vi "CameraSerial_Demo_Legacy.vi"() -> (4 "图像时间戳":u32=16532020 format="%_32g")   [LabVIEW 2015]
uses:
  F:/labview/labview2014 NI/LabVIEW 2015/examples/Instrument IO/Serial/support/Serial - Settings.ctl
  <vilib>/Instr/_visa.llb/VISA Configure Serial Port (Instr).vi
  MVCAMSDK.dll
  <vilib>/Analysis/NI_AALBase.lvlib
panel:
  in  "停止":bool
  out "信号曲线":cluster{dbl[], dbl[]}(graph)
  in  "串口设置":T1={"波特率"=9600, "数据比特"=8, "奇偶"=enum."None", "停止位"=10, "流控制"=0} {"流控制" items=["无"=0, "XON/XOFF"=1, "RTS/CTS"=2, "DTR/DSR"=4]; "停止位" items=["1.0"=10, "1.5"=15, "2.0"=20]; "数据比特" min=5 max=8 step=1; "波特率" items=["75"=75, "110"=110, "134"=134, "150"=150, "300"=300, "600"=600, "1200"=1200, "1800"=1800, "2400"=2400, "4800"=4800, "7200"=7200, "9600"=9600, "14400"=14400, "19200"=19200, "28800"=28800, "38400"=38400, "56000"=56000, "57600"=57600, "115200"=115200, "128000"=128000, "230400"=230400]}
  in  "VISA资源名称":refnum<visa-resource-name>="COM3"
  out "variance 2":dbl caption="方差2" format="%0.3e"
  out "光强图 2":u64[](graph)
  out "variance":dbl caption="方差" format="%0.3e"
  out "相机图像":T2(plugin-control)
  out "光强图":u64[](graph)
  in  "自定义分辨率设置":bool
  in  "预设分辨率设置":bool
  out "帧速":u32
  out "帧间耗时\n单位：（0.1ms）":u32
  in  "相机枚举":T3(ring)
  in  "自动曝光模式":bool=TRUE caption="软触发"
  in  "手动曝光模式":bool caption="软触发"
  in  "硬触发模式":bool caption="软触发"
  in  "软触发模式":bool caption="软触发"
  in  "连续模式":bool caption="软触发"
  in  "软触发一帧":bool caption="软触发"
  in  "读取自定义数据":bool
  in  "写入自定义数据":bool
  in  "拍照":bool
  in  "相机参数":bool=TRUE
  in  "Stop":bool
  in  "激活预览":bool=TRUE
  out "Image":T2(plugin-control)
  # "写入自定义数据"
  # "相机原生分辨率设置"
  # "触发设置"
  # "曝光设置"
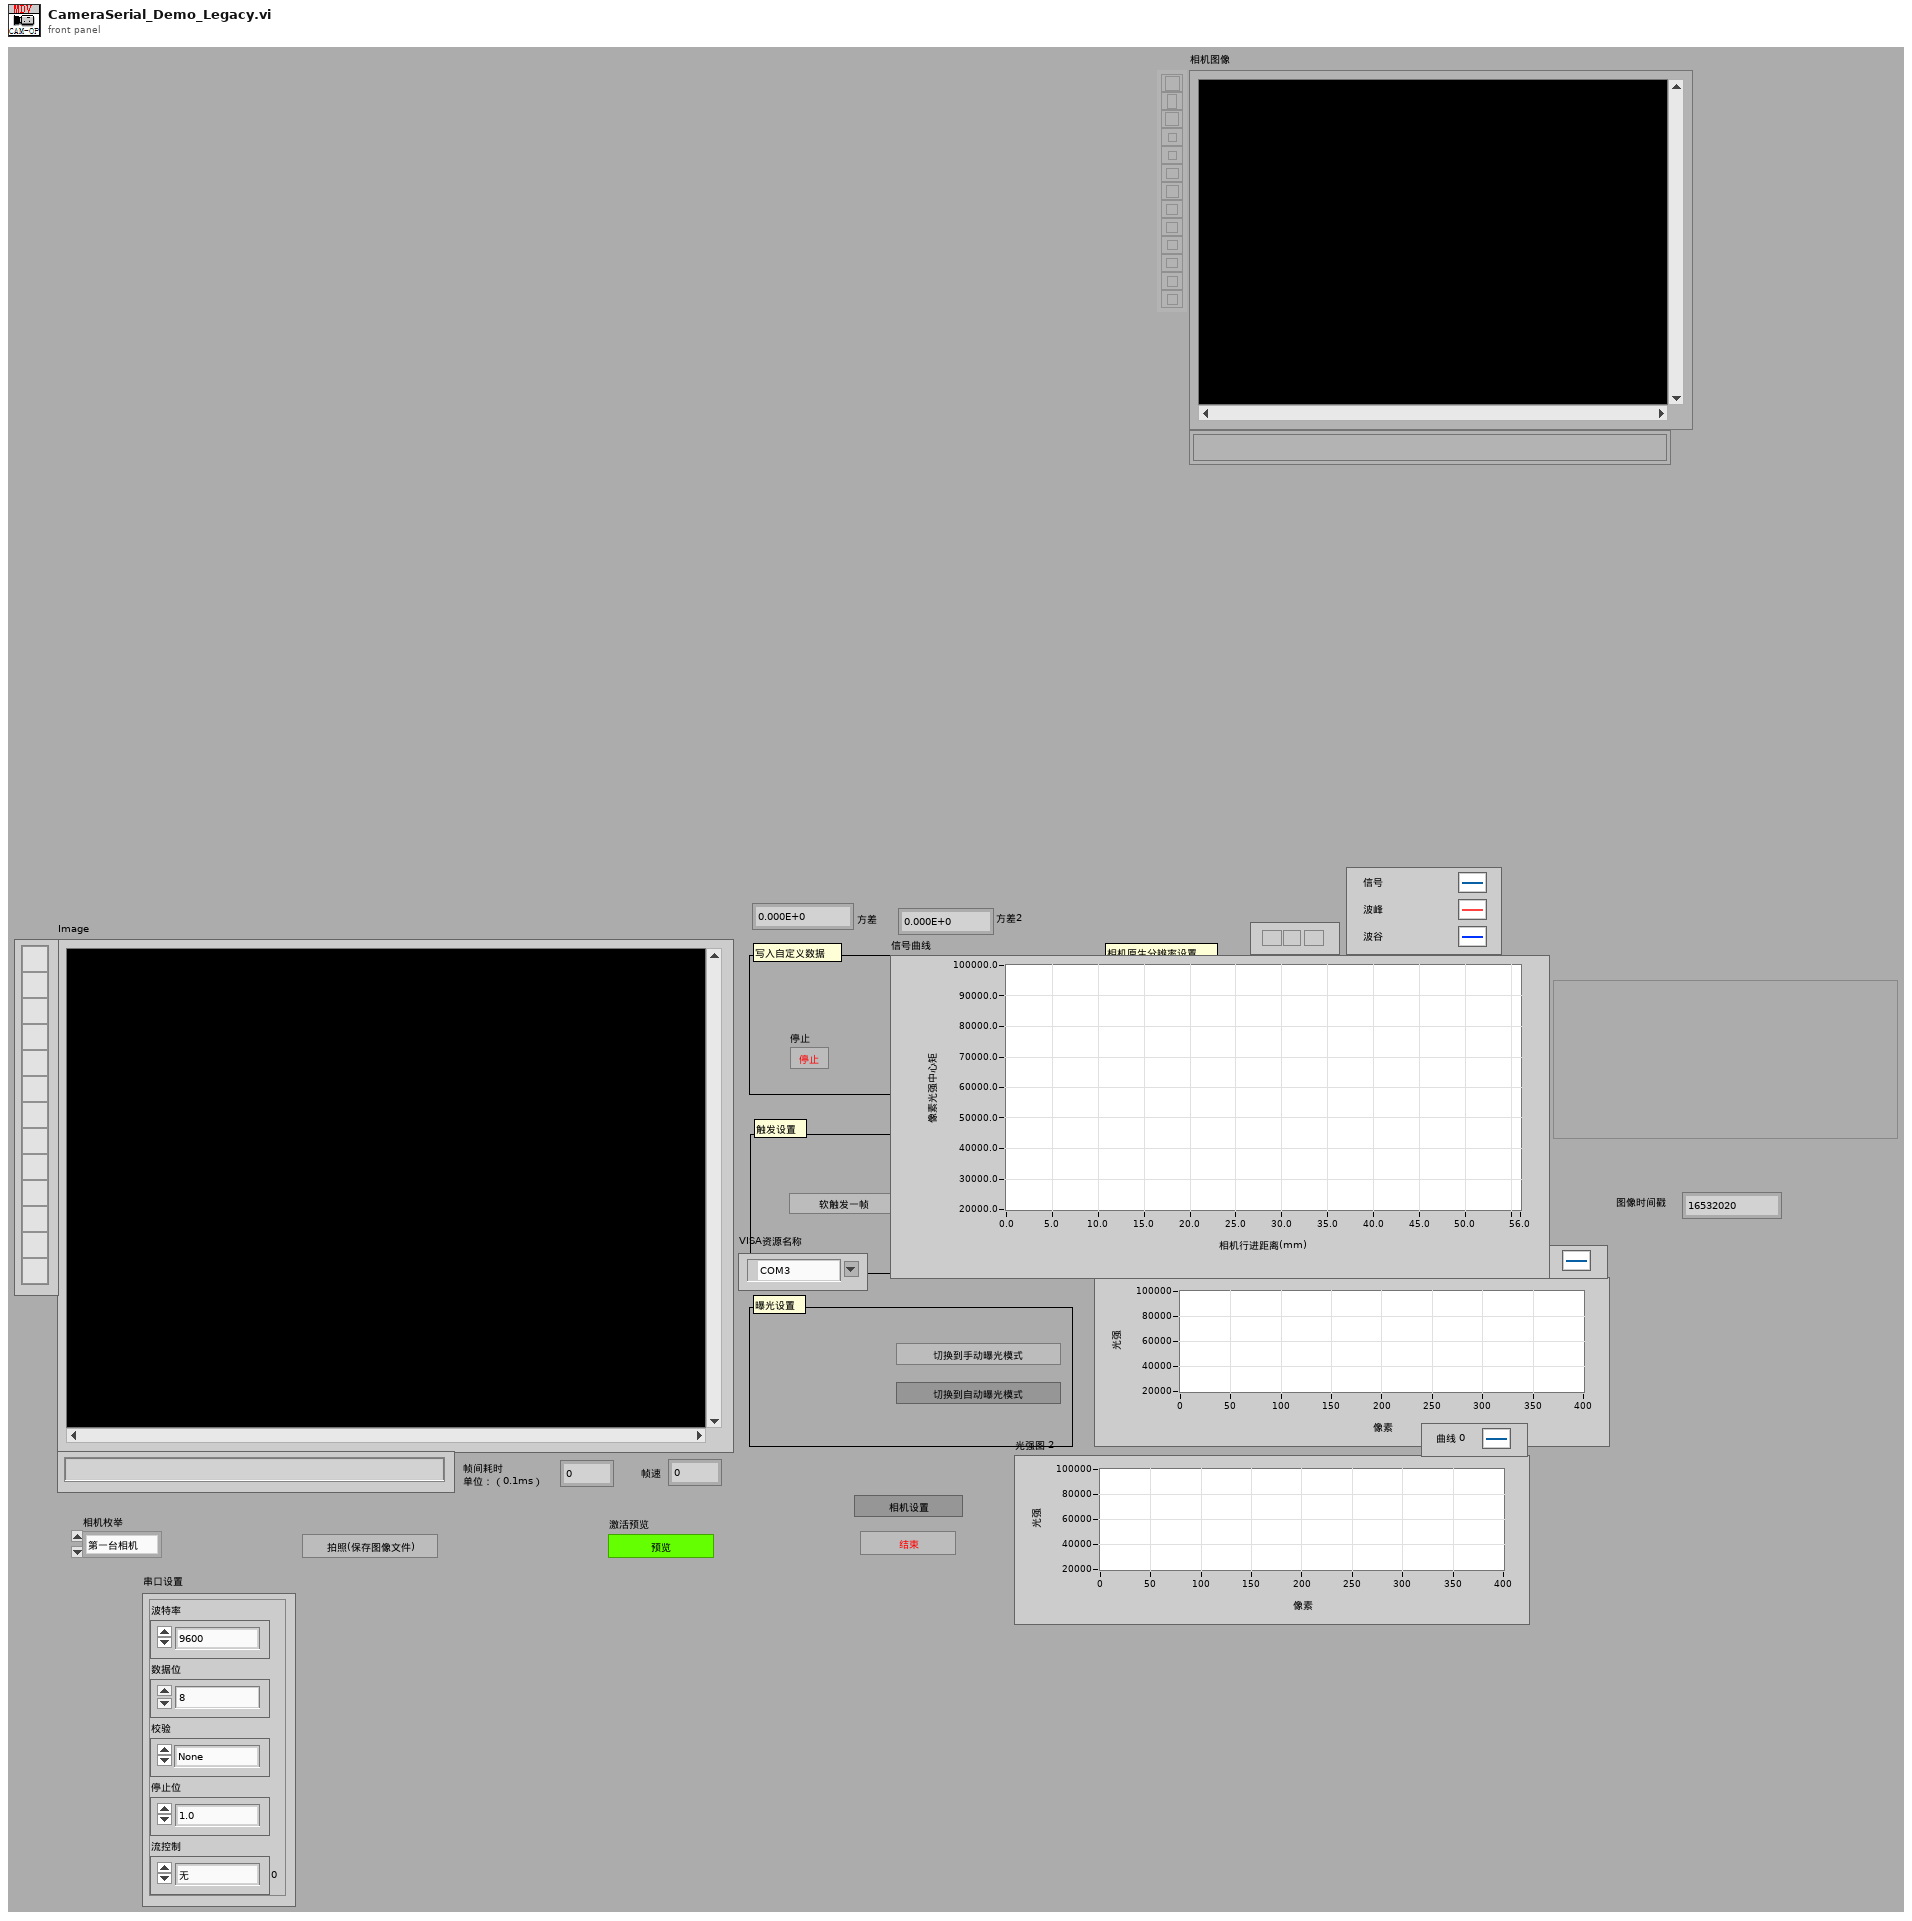
[diagram p1: front panel]
types:
  T1 = typedef "Serial - Settings.ctl" = cluster{"波特率":u32, "数据比特":u16, "奇偶":enum16{"None", "Odd", "Even", "Mark", "Space"}, "停止位":u16, "流控制":u16}
  T2 = typedef "IMAQ Image.ctl" = refnum<image>
  T3 = enum16{"第一台相机", "第二台相机", "第三台相机", "第四台相机", "第五台相机"}
  T4 = typedef "Image Type" = u32
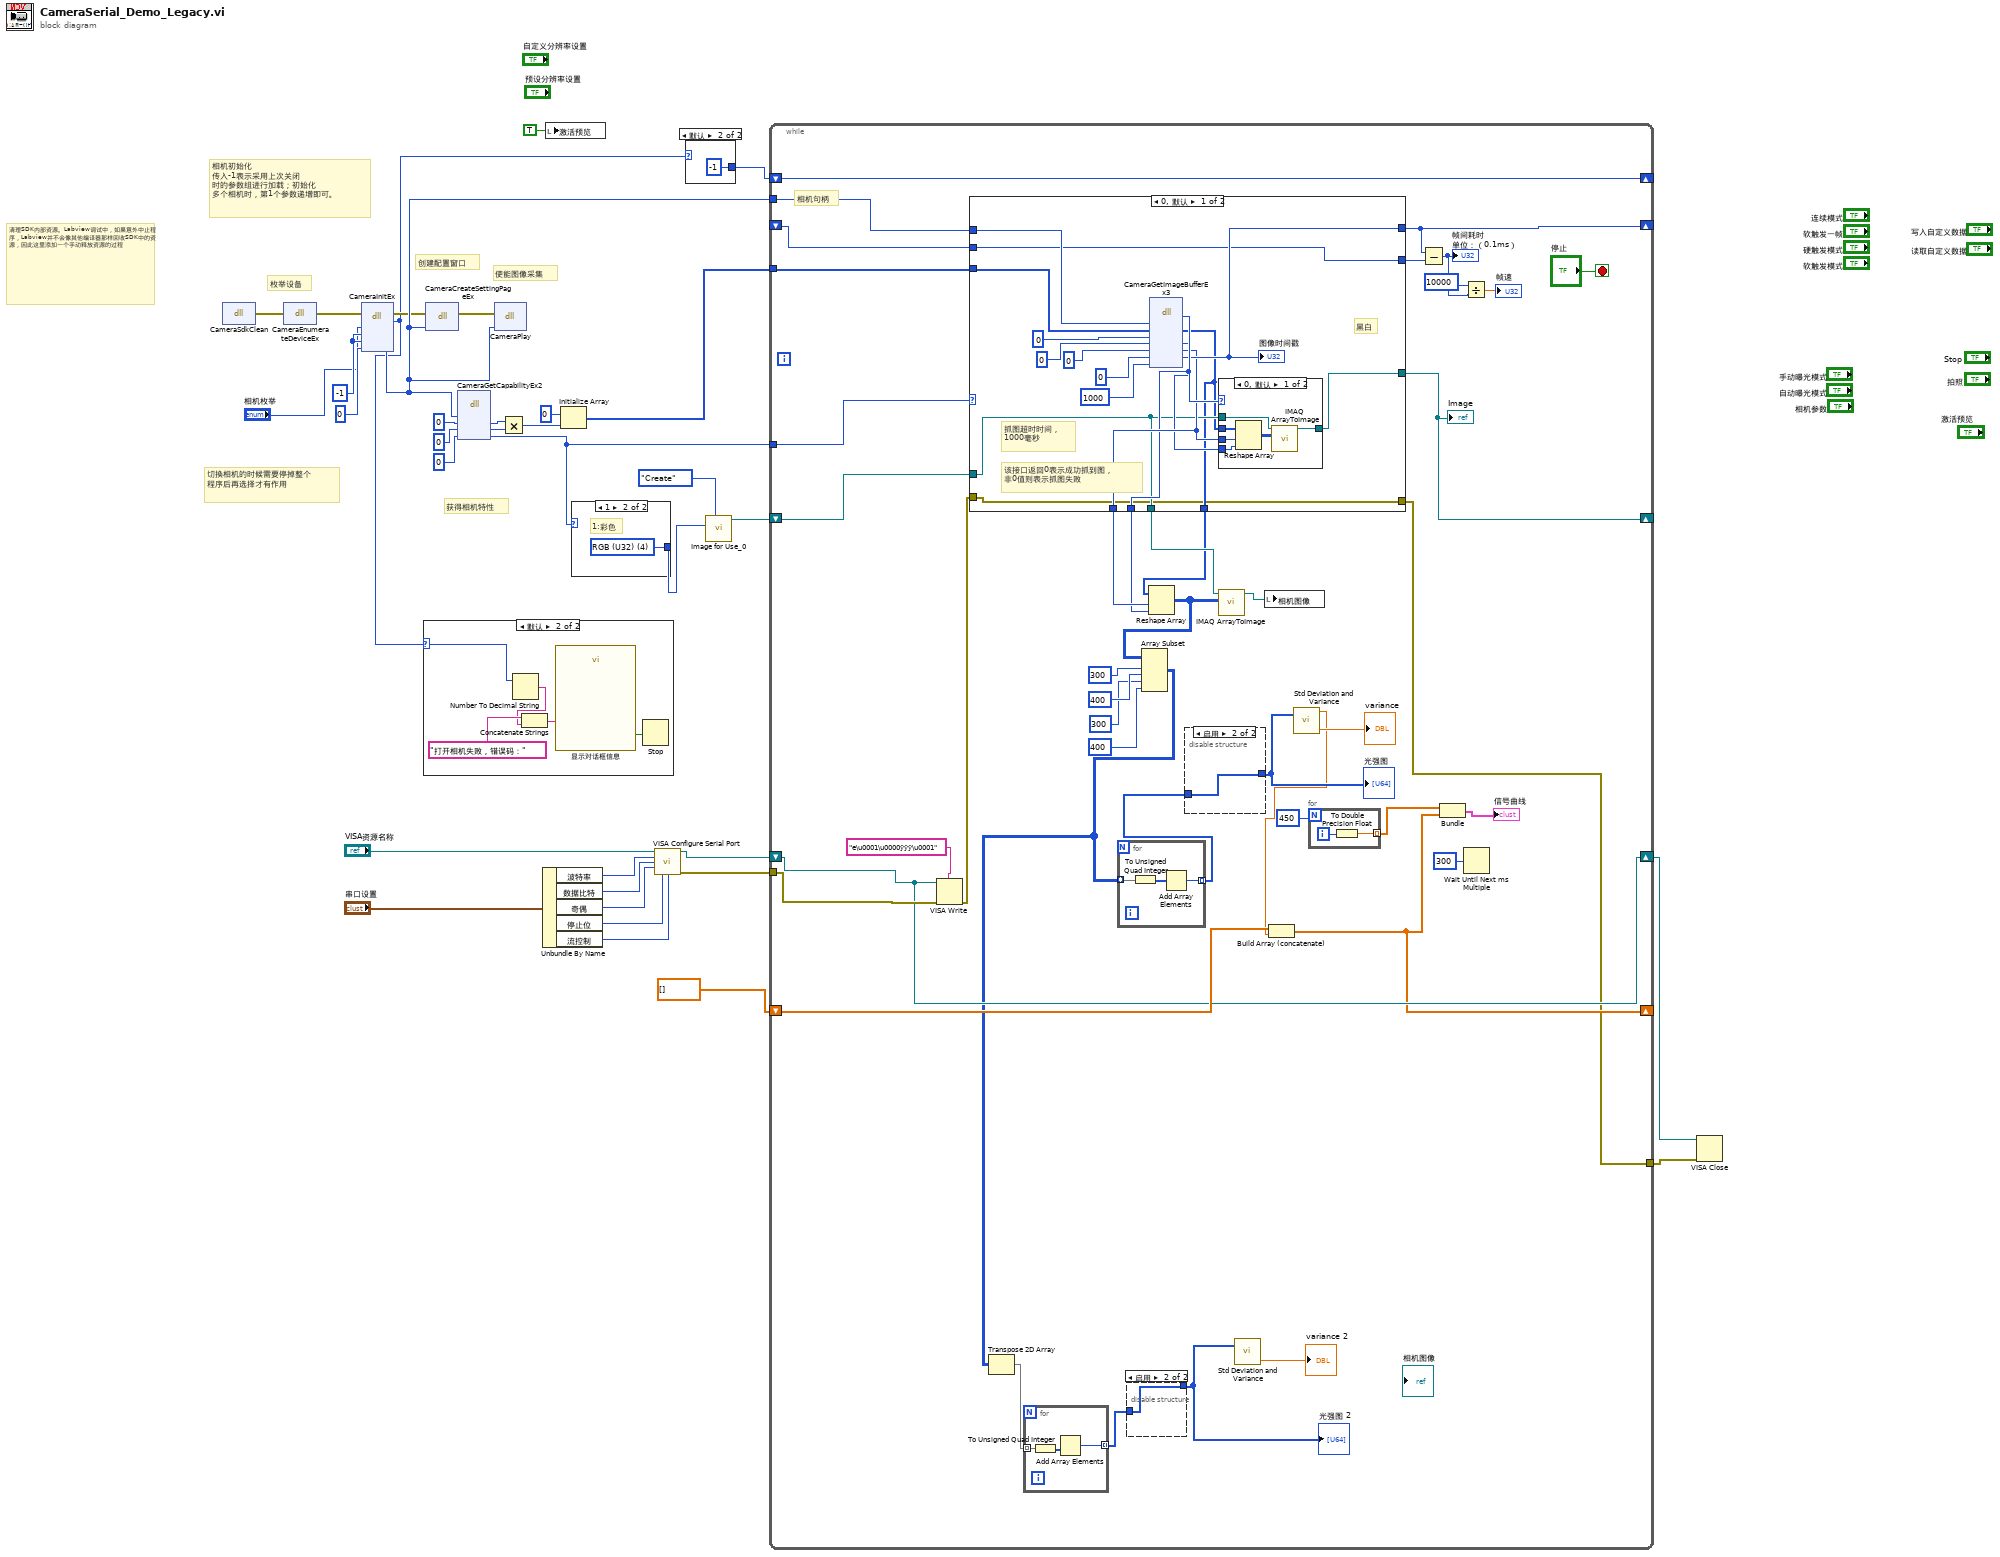
[diagram p0: block diagram]
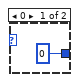
[diagram p2: hidden frame]
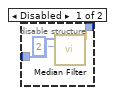
[diagram p4: hidden frame]
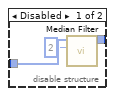
[diagram p5: hidden frame]
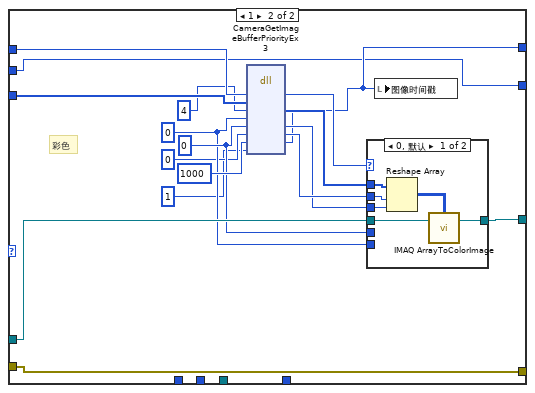
[diagram p7: hidden frame]
diagram:
  w32 = -1
  # "切换相机的时候需要停掉整个\n程序后再选择才有作用"
  # "清理SDK内部资源。Labview调试中，如果意外中止程序，Labview并不会像其他编译器那样回收SDK中的资源，因此这里添加一个手动释放资源的过程"
  # "使能图像采集"
  # "获得相机特性"
  # "创建配置窗口"
  # "相机初始化\n传入-1表示采用上次关闭\n时的参数组进行加载；初始化\n多个相机时，第1个参数递增即可。"
  # "枚举设备"
  n1 = dll-call lib="MVCAMSDK.dll" fn="CameraSdkClean"() -> (error out=w33:errorcluster)  [unwired: 4 in, 1 out]
  n2 = dll-call lib="MVCAMSDK.dll" fn="CameraEnumerateDeviceEx"(error in=w33) -> (error out=w30:errorcluster)  [unwired: 3 in, 1 out]
  n3 = dll-call lib="MVCAMSDK.dll" fn="CameraInitEx"(error in=w30, "相机索引值"="相机枚举", "参数加载方式"=w32, "要加载的参数组索引"=w32, "相机句柄"=0) -> (error out=w19:errorcluster, "返回类型"=w14:i32, "相机句柄"=w21:i32)  [unwired: 5 in, 1 out]
  n4 = case shown="默认" w14 {
    selector: w14 -> [_ w39]
    frame 0 {
    }
    frame Default {
      n5 = Number To Decimal String(number=w39) -> (decimal integer string=w36:string)  [unwired: 1 in]
      n6 = Concatenate Strings("打开相机失败，错误码：" ("字符串"), w36) -> (w38:string)
      n7 = call "显示对话框信息"("Message"=w38) -> ("结束"=w40:bool)  [unwired: 9 in, 1 out]
      n8 = Stop(stop? (T)=w40) -> ()
    }
  }
  n9 = dll-call lib="MVCAMSDK.dll" fn="CameraCreateSettingPageEx"(error in=w19, "相机句柄"=w21) -> (error out=w22:errorcluster)  [unwired: 4 in, 1 out]
  n10 = dll-call lib="MVCAMSDK.dll" fn="CameraGetCapabilityEx2"("相机句柄"=w21, "图像最大宽度"=0, "图像最大高度"=0, "是否是彩色相机(返回0:黑白;1:彩色)"=0) -> ("图像最大宽度"=w24:i32, "图像最大高度"=w23:i32, "是否是彩色相机(返回0:黑白;1:彩色)"=w18:i32)  [unwired: 5 in, 2 out]
  n11 = dll-call lib="MVCAMSDK.dll" fn="CameraPlay"(error in=w22, "相机句柄"=w21) -> ()  [unwired: 4 in, 2 out]
  n12 = Multiply(x=w24, y=w23) -> (x*y=w28:i32)
  n13 = Unbundle By Name("串口设置") -> ("波特率"=w10:u32, "数据比特"=w9:u16, "奇偶"=w8:enum16{"None", "Odd", "Even", "Mark", "Space"}, "停止位"=w7:u16, "流控制"=w6:u16)
  n14 = local write "激活预览"(TRUE ("激活预览")) -> ()
  n15 = Initialize Array(0, w28) -> (w20:i32[])
  n16 = case shown="1" w18 {
    tunnel: [_ w41] -> w34
    frame 0, Default {
      # "0:黑白;"
    }
    frame 1 {
      w41 = T4 4 items=["Grayscale (U8)", "Grayscale (I16)", "Grayscale (SGL)", "Complex (CSG)", "RGB (U32)", "HSL (U32)", "RGB (U64)", "Grayscale (U16)"] ("Image Type")
      # "1:彩色"
    }
  }
  n17 = call-poly "VISA Configure Serial Port"("VISA resource name"="VISA资源名称", "baud rate (9600)"=w10, "data bits (8)"=w9, "parity (0:none)"=w8, "stop bits (10: 1 bit)"=w7, "flow control (0:none)"=w6) -> ("VISA resource name out"=w5:refnum<visa-resource-name>, "error out"=w4:errorcluster)  [unwired: 3 in, 5 out]
  n18 = case shown="默认" w14 {
    tunnel: [0 -1] -> w13
    frame 0 {
    }
    frame Default {
    }
  }
  n19 = call "Image for Use_0.vi"("Command"=enum16{"Create", "Use", "Copy in", "Dispose"}."Create", "Image Type"=w34) -> ("Image out"=w17:T2)  [unwired: 8 in, 1 out]
  n20 = while {
    tunnel: w21 -> [w83]
    tunnel: w20 -> [w85]
    tunnel: w18 -> [w86]
    shift-right: [w82] -> _
    shift-left: w13 -> [w82]
    shift-right: [w81] -> _
    shift-left: w17 -> [w84]
    shift-right: [w80] -> _
    shift-left: _ -> [w79]
    tunnel: w4 -> [w78]
    tunnel: [w73] -> w3
    shift-right: [w76] -> w2
    shift-left: w5 -> [w76]
    shift-right: [w75] -> _
    shift-left: dbl[] [] -> [w77]
    stop <- "停止" stop-if-true
    # "相机句柄"
    n21 = VISA Write(VISA resource name=w76, write buffer="e\u0001\u0000ÿÿÿ\u0001" ("Command"), error in (no error)=w78) -> (error out=w44:errorcluster)  [unwired: 2 out]
    n22 = case shown="0, 默认" w86 {
      tunnel: w85 -> [w118 w142]
      tunnel: w84 -> [w105 w141]
      tunnel: w83 -> [w110 w140]
      tunnel: [w111 w130] -> w81
      tunnel: [w109 w129] -> w80
      tunnel: w79 -> [w108 w128]
      tunnel: [w108 w128] -> w72
      tunnel: [w107 _] -> w66
      tunnel: [w106 _] -> w65
      tunnel: [w105 _] -> w64
      tunnel: [w104 _] -> w63
      tunnel: w44 -> [w103 w126]
      tunnel: [w103 w126] -> w73
      frame 0, Default {
        # "黑白"
        # "该接口返回0表示成功抓到图，\n非0值则表示抓图失败"
        # "抓图超时时间，\n1000毫秒"
        n23 = dll-call lib="MVCAMSDK.dll" fn="CameraGetImageBufferEx3"("相机句柄"=w110, "图像数据缓冲区"=w118, "图像输出格式(0:8位灰度;1:24位彩色;2:32位彩色，3：BGR24彩色 4：BGRA32位彩色)"=0, "图像宽度"=0, "图像高度"=0, "时间戳(单位为100微秒)"=0, "抓图超时时间(毫秒)"=1000) -> ("返回类型"=w113:i32, "图像数据缓冲区"=w104:u8[], "图像宽度"=w106:i32, "图像高度"=w107:i32, "时间戳(单位为100微秒)"=w109:u32)  [unwired: 6 in, 2 out]
        "图像时间戳" <- w109
        n24 = case shown="0, 默认" w113 {
          tunnel: w104 -> [w124 _]
          tunnel: w105 -> [w121 w125]
          tunnel: w107 -> [w123 _]
          tunnel: w106 -> [w122 _]
          tunnel: [w119 w125] -> w111
          frame 0, Default {
            n25 = Reshape Array(w124, w123, w122) -> (w120:u8[][])
            n26 = call "IMAQ ArrayToImage"("Image Pixels (U8)"=w120, "Image"=w121) -> ("Image Out"=w119:T2)  [unwired: 8 in, 1 out]
          }
          frame -12 {
          }
        }
      }
      frame 1 {
        w132 = 0
        w133 = 0
        # "彩色"
        n27 = dll-call lib="MVCAMSDK.dll" fn="CameraGetImageBufferPriorityEx3"("相机句柄"=w140, "图像数据缓冲区"=w142, "图像输出格式(0:8位灰度;1:24位彩色;2:32位彩色)"=4, "图像宽度"=w132, "图像高度"=w133, "时间戳（单位为100微秒）"=0, "抓图超时时间(毫秒)"=1000, "取图优先级(0: 取最旧   1:取最新)"=1) -> ("返回类型"=w134:i32, "图像数据缓冲区"=w137:u32[], "图像宽度"=w135:i32, "图像高度"=w136:i32, "时间戳（单位为100微秒）"=w129:u32)  [unwired: 7 in, 2 out]
        n28 = case shown="0, 默认" w134 {
          tunnel: w137 -> [w147 _]
          tunnel: w141 -> [w146 w149]
          tunnel: w136 -> [w145 _]
          tunnel: w135 -> [w144 _]
          tunnel: w133 -> [_ _]
          tunnel: w132 -> [_ _]
          tunnel: [w143 w149] -> w130
          frame 0, Default {
            n29 = Reshape Array(w147, w145, w144) -> (w148:u32[][])
            n30 = call "IMAQ ArrayToColorImage"("Image Pixels (U32)"=w148, "Image"=w146) -> ("Image Out"=w143:T2)  [unwired: 3 in, 1 out]
          }
          frame -12 {
          }
        }
        n31 = local write "图像时间戳"(w129) -> ()
      }
    }
    "Image" <- w81
    n32 = Reshape Array(w63, w66, w65) -> (w51:u8[][])
    n33 = Array Subset(array=w51, index (row)=300 ("索引"), length (row)=400 ("长度"), index (col)=300 ("长度"), length (col)=400 ("索引")) -> (w50:u8[][])
    n34 = Transpose 2D Array(2D array=w50) -> (transposed array=w58:u8[][])
    n35 = for {
      tunnel: w58 -> [w90] mode=indexing
      tunnel: [w91] -> w59 mode=indexing
      n36 = To Unsigned Quad Integer(1:w90) -> (0:w89:u64[])
      n37 = Add Array Elements(numeric array=w89) -> (sum=w91:u64)
    }
    n38 = for {
      tunnel: w50 -> [w97] mode=indexing
      tunnel: [w98] -> w61 mode=indexing
      n39 = To Unsigned Quad Integer(1:w97) -> (0:w96:u64[])
      n40 = Add Array Elements(numeric array=w96) -> (sum=w98:u64)
    }
    n41 = disable-structure shown="启用" {
      disable-tunnel: w59 -> [w94 w95]
      disable-tunnel: [w92 w95] -> w56
      frame Disabled {
        n42 = call <vilib>:"Median Filter.vi"("left rank"=2, "X"=w94) -> ("Filtered X"=w92:dbl[])  [unwired: 8 in, 1 out]
      }
      frame Enabled {
      }
    }
    "光强图 2" <- w56
    n43 = disable-structure shown="启用" {
      disable-tunnel: w61 -> [w101 w102]
      disable-tunnel: [w99 w102] -> w57
      frame Disabled {
        n44 = call <vilib>:"Median Filter.vi"("left rank"=2, "X"=w101) -> ("Filtered X"=w99:dbl[])  [unwired: 8 in, 1 out]
      }
      frame Enabled {
      }
    }
    "光强图" <- w57
    n45 = call "IMAQ ArrayToImage"("Image Pixels (U8)"=w51, "Image"=w64) -> ("Image Out"=w67:T2)  [unwired: 8 in, 1 out]
    n46 = call <vilib>:"Std Deviation and Variance.vi"("X"=w56) -> ("variance"=→"variance 2":dbl)  [unwired: 1 in, 2 out]
    n47 = local write "相机图像"(w67) -> ()
    n48 = call <vilib>:"Std Deviation and Variance.vi"("X"=w57) -> ("mean"=w46:dbl, "variance"=→"variance":dbl)  [unwired: 1 in, 1 out]
    n49 = Build Array (concatenate)(w77, w46) -> (w75:dbl[])
    n50 = for {
      N: 450 -> [_]
      tunnel: [w87] -> w48 mode=indexing
      i -> [w88]
      n51 = To Double Precision Float(number=w88) -> (double precision float=w87:dbl)
    }
    n52 = Subtract(x=w80, y=w72) -> (x-y=w71:u32)
    "帧间耗时\n单位：（0.1ms）" <- w71
    n53 = Bundle(w48, w75) -> (→"信号曲线":cluster{dbl[], dbl[]})  [unwired: 1 in]
    n54 = Divide(x=u32 10000 ("帧间耗时"), y=w71) -> (x/y=→"帧速":dbl)
    n55 = Wait Until Next ms Multiple(millisecond multiple=u32 300 ("毫秒倍数")) -> ()  [unwired: 1 out]
  }
  n56 = VISA Close(VISA resource name=w2, error in (no error)=w3) -> ()  [unwired: 1 out]
